vi "ConcatenateZones.vi"(8 "error in (no error)":errorcluster, 11 "Zone in":refnum<class "Zone.lvclass">) -> (0 "error out":errorcluster, 3 "Zone out":refnum<class "Zone.lvclass">)   [LabVIEW 2023, in "Zone.lvclass"]
uses:
  Zone.lvclass
panel:
  in  "Zone to Add":refnum<class "Zone.lvclass">
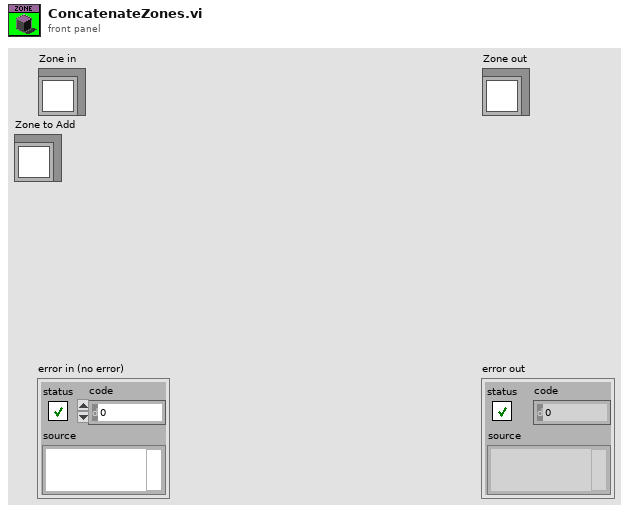
[diagram p1: front panel]
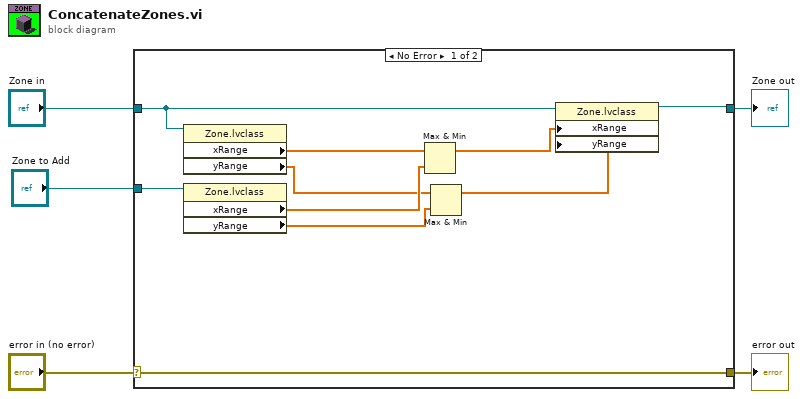
[diagram p0: block diagram]
diagram:
  n1 = case shown="No Error" "error in (no error)" {
    selector: "error in (no error)" -> [w15 w17]
    tunnel: [w15 w17] -> w4
    tunnel: [w8 w16] -> w2
    tunnel: "Zone in" -> [w9 w16]
    tunnel: "Zone to Add" -> [w14 _]
    frame No Error {
      n2 = property class="Zone.lvclass"(reference=w9) -> ("xRange"=w13:dbl[], "yRange"=w11:dbl[])  [unwired: 1 in, 2 out]
      n3 = property class="Zone.lvclass"(reference=w14) -> ("xRange"=w12:dbl[], "yRange"=w10:dbl[])  [unwired: 1 in, 2 out]
      n4 = Max & Min(x=w13, y=w12) -> (max(x,y)=w7:dbl[])  [unwired: 1 out]
      n5 = Max & Min(x=w11, y=w10) -> (max(x,y)=w6:dbl[])  [unwired: 1 out]
      n6 = property class="Zone.lvclass"(reference=w9, "xRange"=w7, "yRange"=w6) -> (reference out=w8:refnum<class "Zone.lvclass">)  [unwired: 1 in, 1 out]
    }
    frame Error {
    }
  }
  "error out" <- w4
  "Zone out" <- w2
